vi "remote.Disconnect.vi"(0 "SLSC Remote in":refnum<class "SLSC Interface.lvclass">, 5 "devices":refnum<k21>="$DefaultDevices", 11 "error in (no error)":errorcluster) -> (4 "SLSC Remote out":refnum<class "SLSC Interface.lvclass">, 15 "error out":errorcluster)   [LabVIEW 2016, in "SLSC Interfaces.lvlib" / "SLSC Interface.lvclass"]
uses:
  SLSC Interface Class/SLSC Interface.lvclass
  SLSC Interface Class/SLSC Interface.lvclass/SLSC Interface.ctl
  SLSC Interface Class/Read client handle.vi
  SLSC Interface Class/Read URL.vi
  <vilib>/NI/JSON Support for LabVIEW/JSON Data Classes/JSON Object/JSON Object.lvclass
  C:/Program Files (x86)/National Instruments/LabVIEW 2016/vi.lib/NI/JSON Support for LabVIEW/JSON Data Classes/JSON Datatype/JSON Null.lvclass
  SLSC Interface Class/Read session.vi
  <vilib>/NI/JSON Support for LabVIEW/JSON Data Classes/JSON Object/New JSON Object (Empty).vi
  <vilib>/NI/JSON Support for LabVIEW/JSON Data Classes/JSON Object/Insert Key Value Pair (Single String).vi
  <vilib>/NI/NI JSONRPC Server Framework/Classes/Server/Format Client Request (Auto-Increment).vi
  <vilib>/httpClient/POSTBuffer.vi
  <vilib>/NI/NI JSONRPC Server Framework/Classes/Server/Parse Response (Object).vi
  <vilib>/NI/NI JSONRPC Server Framework/Classes/Server/JSONRPC Server.lvclass
  <vilib>/httpClient/LabVIEWHTTPClient.lvlib
  <vilib>/NI/JSON Support for LabVIEW/JSON Data Classes/JSON Helper/JSON Helper.lvclass
  C:/Program Files (x86)/National Instruments/LabVIEW 2016/vi.lib/NI/JSON Support for LabVIEW/JSON Data Classes/JSON Structured Type/JSON Structure.lvclass
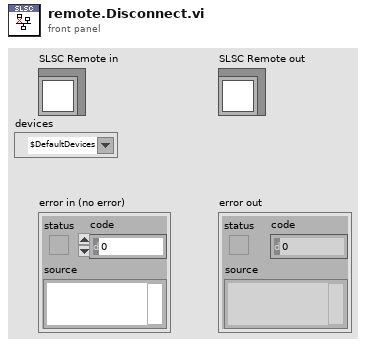
[diagram p1: front panel]
types:
  T1 = typedef "LabVIEWHTTPClient.lvlib/ClientHandle.ctl" = refnum<k1>
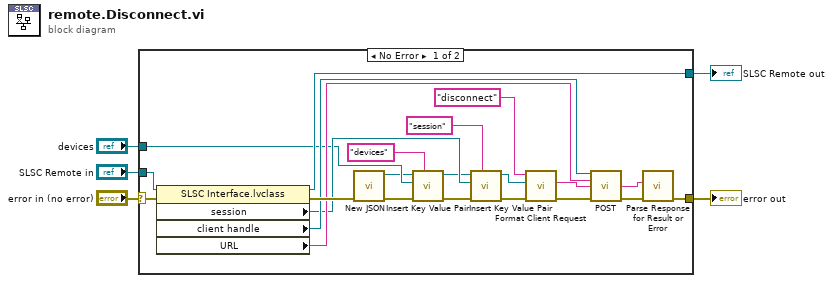
[diagram p0: block diagram]
diagram:
  n1 = case shown="No Error" "error in (no error)" {
    selector: "error in (no error)" -> [w25 w28]
    tunnel: "devices" -> [w10 _]
    tunnel: "SLSC Remote in" -> [w27 w29]
    tunnel: [w26 w29] -> w4
    tunnel: [w12 w28] -> w2
    frame No Error {
      n2 = property class="SLSC Interface.lvclass"(reference=w27, error in=w25) -> (reference out=w26:refnum<class "SLSC Interface.lvclass">, error out=w24:errorcluster, "session"=w11:refnum<k21>, "client handle"=w17:T1, "URL"=w16:string)
      n3 = call-poly <vilib>:"New JSON.vi"("error in (no error)"=w24) -> ("error out"=w23:errorcluster, "JSON Object out"=w9:refnum<class "JSON Object.lvclass">)  [unwired: 9 in]
      n4 = call-poly <vilib>:"Insert Key Value Pair.vi"("key"="devices" ("Name"), "error in (no error)"=w23, "value"=w10, "JSON Object in"=w9) -> ("error out"=w22:errorcluster, "JSON Object out"=w8:refnum<class "JSON Object.lvclass">)  [unwired: 5 in, 1 out]
      n5 = call-poly <vilib>:"Insert Key Value Pair.vi"("key"="session" ("Name"), "error in (no error)"=w22, "value"=w11, "JSON Object in"=w8) -> ("error out"=w18:errorcluster, "JSON Object out"=w19:refnum<class "JSON Object.lvclass">)  [unwired: 5 in, 1 out]
      n6 = call-poly <vilib>:"Format Client Request.vi"("error in (no error)"=w18, "JSON in"=w19, "method"="disconnect") -> ("error out"=w15:errorcluster, "Request String"=w20:string)  [unwired: 7 in]
      n7 = call-poly <vilib>:"POST.vi"("client handle"=w17, "url"=w16, "buffer"=w20, "error in (no error)"=w15) -> ("body"=w14:string, "error out"=w13:errorcluster)  [unwired: 8 in, 2 out]
      n8 = call-poly <vilib>:"Parse Response for Result or Error.vi"("error in"=w13, "Response String In"=w14) -> ("error out"=w12:errorcluster)  [unwired: 7 in, 2 out]
    }
    frame Error {
    }
  }
  "error out" <- w2
  "SLSC Remote out" <- w4
